vi "ITX_Global.vi"() -> ()   [LabVIEW 2011]
panel:
  in  "PPMS T & B log file":path=path "C:/Users/PPMS/Log/LogB_T.dat"
  in  "pickering path":path=path "C:/LabView/PPMS basic VIs/Switch Status.txt"
  in  "image path":path=path "C:/Experiments/2011-summer Superconductivity-Spin Hall/Device images/SA02522N.20120611.png"
  in  "filename":string="SA02650"
  in  "path":path=path "C:/Users/Mengchen/20121207 LAO_STO_SiC/SA02650 LAO_STO_SiC add"
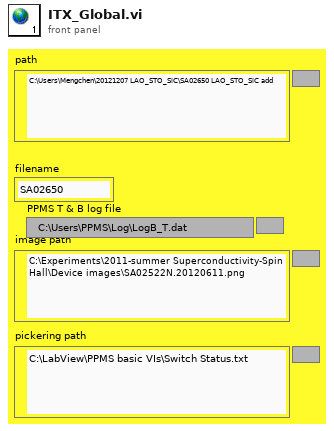
[diagram p1: front panel]
diagram:
